vi "[FPGA] Load and PV controller_9039.vi"() -> ()   [LabVIEW 2015]
uses:
  <vilib>/rvi/Emulation/niFpgaGetClockAttributes.vi
  <vilib>/rvi/Emulation/niFpgaSctlEmulationGetInTimedLoop.vi
  <vilib>/rvi/Emulation/niFpgaEmulationReportErrorSimple.vi
  <vilib>/rvi/eio/common/nirviEmuTemplateMethod_errors.vi
  <vilib>/rvi/Emulation/niFpgaCriticalErrorInLSC.vi
  <vilib>/eio/EIONode/EIONode.xnode
panel:
  in  "PV Relay closed":bool
  out "Loop dT (Ticks)":u32=3000
  in  "Loop Rate (Ticks)":u32=1000
  in  "Load Relay closed":bool
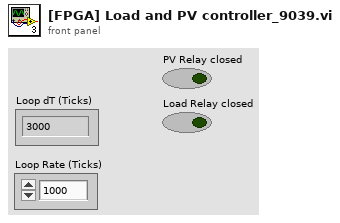
[diagram p1: front panel]
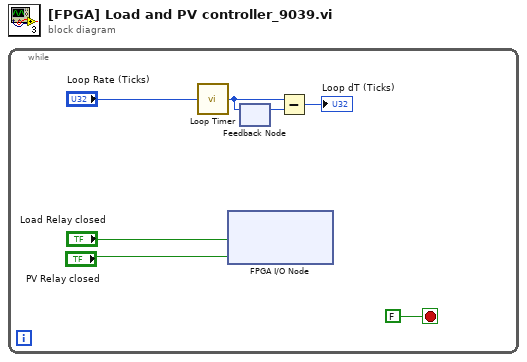
[diagram p0: block diagram]
diagram:
  n1 = while {
    stop <- FALSE ("stop") stop-if-true
    n2 = call "Loop Timer"("Count(Ticks)"="Loop Rate (Ticks)") -> ("Tick Count(Ticks)"=w5:u32)
    n3 = xnode "FPGA I/O Node"("Mod1/DIO0"="Load Relay closed", "Mod1/DIO1"="PV Relay closed") -> ()  [unwired: 2 in, 2 out]
    n4 = feedback #1() -> (w6:u32)  [unwired: 1 in]
    n5 = feedback-in #1(w5) -> ()
    n6 = Subtract(x=w5, y=w6) -> (x-y=→"Loop dT (Ticks)":u32)
  }
